vi "Get Target Item.vi"(8 "error in (no error)":errorcluster, 11 "Builder in":refnum<class "Builder.lvclass">) -> (0 "error out":errorcluster, 3 "Builder out":refnum<class "Builder.lvclass">)   [LabVIEW 2019, in "Builder.lvclass"]
uses:
  Builder/Builder.lvclass
  Builder/Builder.lvclass/Builder.ctl
  <vilib>/Utility/error.llb/Error Cluster From Error Code.vi
  <vilib>/ErrorRing/Error Ring.xnode
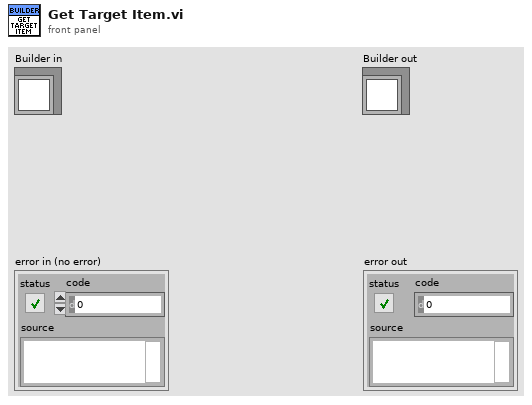
[diagram p1: front panel]
types:
  T1 = typedef "TargetType.ctl" = enum16{"Windows", "cRIO-9045"}
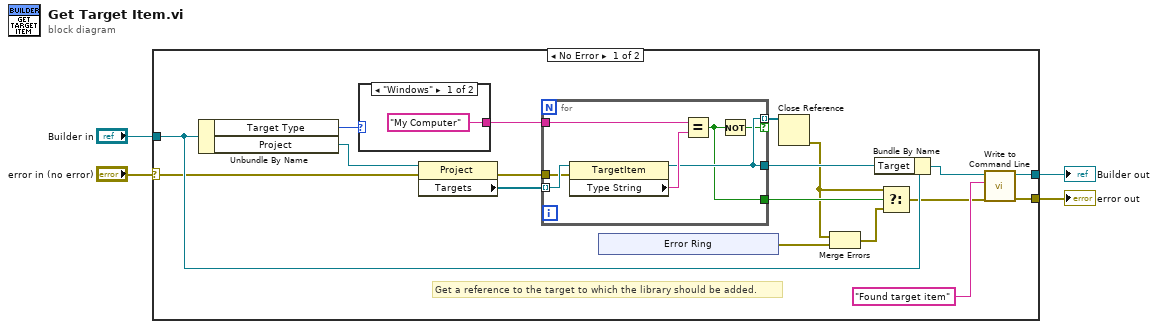
[diagram p0: block diagram]
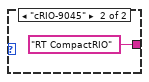
[diagram p2: hidden frame]
diagram:
  n1 = case shown="No Error" "error in (no error)" {
    selector: "error in (no error)" -> [w14 w37]
    tunnel: "Builder in" -> [w15 w36]
    tunnel: [w13 w37] -> w3
    tunnel: [w11 w36] -> w2
    frame No Error {
      # "Get a reference to the target to which the library should be added."
      n2 = Unbundle By Name(w15) -> ("Target Type"=w17:T1, "Project"=w18:refnum<vi>)
      n3 = case shown="\"Windows\"" w17 {
        tunnel: ["My Computer" "RT CompactRIO"] -> w21
        frame "Windows" {
        }
        frame "cRIO-9045" {
        }
      }
      n4 = property class="Project"(reference=w18, error in=w14) -> (error out=w20:errorcluster, "Targets"=w19:refnum<vi>[])  [unwired: 1 out]
      n5 = for {
        tunnel: w19 -> [w35] mode=indexing
        tunnel: w20 -> [w34]
        tunnel: w21 -> [w32]
        tunnel: [w31] -> w16
        tunnel: [w29] -> w9
        tunnel: [w31] -> w22 mode=indexing if=w30
        n6 = property class="TargetItem"(reference=w35, error in=w34) -> (reference out=w31:refnum<vi>, "Type String"=w33:string)  [unwired: 1 out]
        n7 = Equal?(x=w32, y=w33) -> (x = y?=w29:bool)
        n8 = Not(x=w29) -> (.not. x?=w30:bool)
      }
      n9 = xnode "Error Ring"() -> ("error out"=w7:errorcluster)
      n10 = Close Reference(reference=w22) -> (error out=w6:errorcluster)  [unwired: 1 in]
      n11 = Merge Errors(w6, w7) -> (w8:errorcluster)
      n12 = Bundle By Name(cluster=w15, "Target"=w16) -> (w12:refnum<class "Builder.lvclass">)
      n13 = Select(t=w6, s=w9, f=w8) -> (s? t:f=w5:errorcluster)
      n14 = call "Write to Command Line.vi"("error in (no error)"=w5, "Message"="Found target item" ("Text to Write"), "Builder in"=w12) -> ("error out"=w13:errorcluster, "Builder out"=w11:refnum<class "Builder.lvclass">)  [unwired: 7 in]
    }
    frame Error {
    }
  }
  "error out" <- w3
  "Builder out" <- w2
